vi "Configure Trigger Normal.vi"(8 "error in (no error)":errorcluster, 9 "Trigger Delay (0 s)":dbl, 10 "Trigger Hold-off (1E-6 s)":dbl=1e-06, 11 "VISA resource name":refnum<visa-resource-name>) -> (0 "error out":errorcluster, 3 "VISA resource name out":refnum<visa-resource-name>)   [LabVIEW 2018, in "Agilent U2000 Series.lvlib"]
doc: "Configures trigger hold-off and trigger delay for normal measurement.\n\nNote:\nThis VI is only available in Normal measurement mode. You can call <b>Configure Measurement.vi</b> to change the measurement mode."
uses:
  Agilent U2000 Series.lvlib
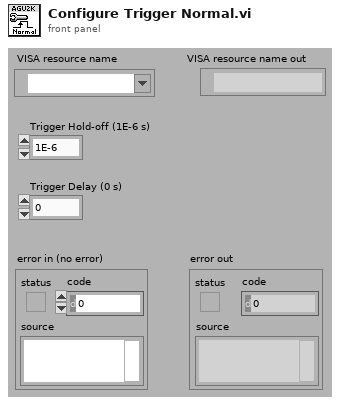
[diagram p1: front panel]
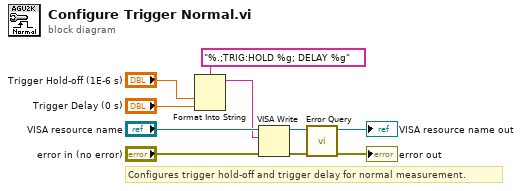
[diagram p0: block diagram]
diagram:
  # "Configures trigger hold-off and trigger delay for normal measurement."
  n1 = Format Into String(format string="%.;TRIG:HOLD %g; DELAY %g", "Trigger Hold-off (1E-6 s)", "Trigger Delay (0 s)") -> (resulting string=w6:string)  [unwired: 2 in, 1 out]
  n2 = VISA Write(VISA resource name="VISA resource name", write buffer=w6, error in (no error)="error in (no error)") -> (VISA resource name out=w3:refnum<visa-resource-name>, error out=w4:errorcluster)  [unwired: 1 out]
  n3 = call "Error Query.vi"("error in (no error)"=w4, "VISA resource name"=w3) -> ("error out"=→"error out":errorcluster, "VISA resource name out"=→"VISA resource name out":refnum<visa-resource-name>)  [unwired: 8 out]
